vi "Write Samples 2.vi"(8 "error in (no error)":errorcluster, 10 "Samples":map{string, refnum<class "Sample.lvclass">}(c390), 11 "Metric in":refnum<class "Metric.lvclass">) -> (0 "error out":errorcluster, 3 "Metric out":refnum<class "Metric.lvclass">)   [LabVIEW 2020, in "Metrics.lvlib" / "Metric.lvclass"]
uses:
  Metric.lvclass
  sample/Sample.lvclass
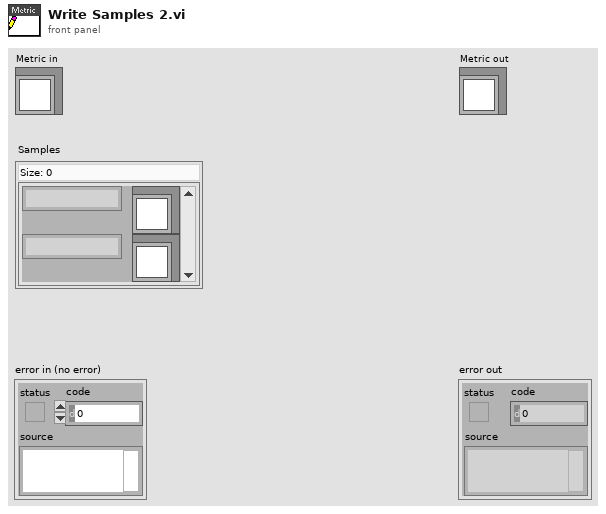
[diagram p1: front panel]
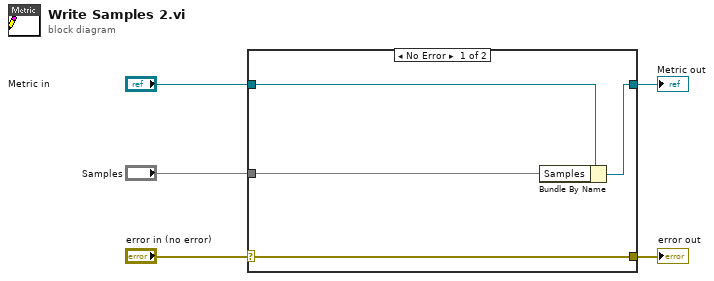
[diagram p0: block diagram]
diagram:
  n1 = case shown="No Error" "error in (no error)" {
    selector: "error in (no error)" -> [w9 w10]
    tunnel: [w9 w10] -> w4
    tunnel: [w7 w11] -> w2
    tunnel: "Metric in" -> [w8 w11]
    tunnel: "Samples" -> [w6 _]
    frame No Error {
      n2 = Bundle By Name(cluster=w8, "Samples"=w6) -> (w7:refnum<class "Metric.lvclass">)
    }
    frame Error {
    }
  }
  "error out" <- w4
  "Metric out" <- w2
